vi "Populate VS channel control- Output Value.vi"(7 "DisplayFilter":u8(ring)=7 items=["K_CHAN_R", "K_CHAN_W", "K_CHAN_RW", "K_CHAN_VOLT", "K_CHAN_FAULT", "K_ALL", "K_CUSTOM", "K_CHAN_R_VIS", "K_CHAN_W_VIS", "K_CHAN_RW_VIS", "K_CHAN_VOLT_VIS", "K_CHAN_FAULT_VIS"], 8 "error in (no error)":errorcluster, 9 "Data cluster in":T1, 10 "NIVS.System Definition Root":refnum<k24>, 11 ".NET Refnum in":refnum<k24>) -> (0 "error out":errorcluster, 3 ".NET Refnum out":refnum<k24>)   [LabVIEW 2013]
uses:
  PWM Object Parameters.ctl
  NationalInstruments.VeriStand.SystemStorageUI
  NationalInstruments.VeriStand.SystemStorage
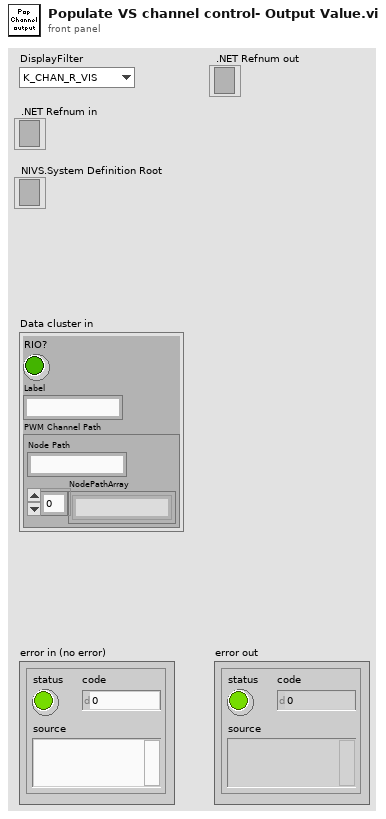
[diagram p1: front panel]
types:
  T1 = typedef "PWM Object Parameters.ctl" = cluster{"RIO?":bool, "Label":string, "PWM Channel Path":cluster{"NodePathArray":string[], "Node Path":string}}
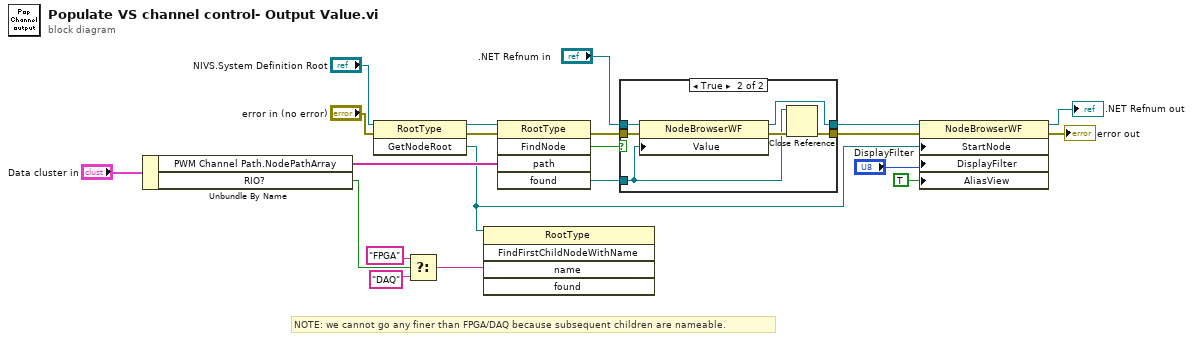
[diagram p0: block diagram]
diagram:
  # "NOTE: we cannot go any finer than FPGA/DAQ because subsequent children are nameable."
  n1 = Unbundle By Name("Data cluster in") -> ("PWM Channel Path.NodePathArray"=w2:string[], "RIO?"=w6:bool)
  n2 = invoke class="RootType" method="GetNodeRoot"(reference="NIVS.System Definition Root", error in="error in (no error)") -> (reference out=w10:refnum<k24>, error out=w9:errorcluster, "GetNodeRoot"=w1:refnum<k24>)  [unwired: 1 in]
  n3 = Select(t="FPGA", s=w6, f="DAQ") -> (s? t:f=w5:string)
  n4 = invoke class="RootType" method="FindFirstChildNodeWithName"(reference=w1, "name"=w5) -> ()  [unwired: 3 in, 5 out]
  n5 = invoke class="RootType" method="FindNode"(reference=w10, error in=w9, "path"=w2) -> (error out=w16:errorcluster, "FindNode"=w18:bool, "found"=w15:refnum<k24>)  [unwired: 2 in, 2 out]
  n6 = case shown="True" w18 {
    tunnel: w15 -> [_ w24]
    tunnel: w16 -> [w23 w25]
    tunnel: [w23 w28] -> w17
    tunnel: ".NET Refnum in" -> [w22 w27]
    tunnel: [w22 w26] -> w19
    frame False {
    }
    frame True {
      n7 = property class="NodeBrowserWF"(reference=w27, error in=w25, "Value"=w24) -> (reference out=w26:refnum<k24>, error out=w29:errorcluster)
      n8 = Close Reference(reference=w24, error in (no error)=w29) -> (error out=w28:errorcluster)
    }
  }
  n9 = property class="NodeBrowserWF"(reference=w19, error in=w17, "StartNode"=w1, "DisplayFilter"="DisplayFilter", "AliasView"=TRUE) -> (reference out=→".NET Refnum out":refnum<k24>, error out=→"error out":errorcluster)
